vi "DCC_set_mode.vi"(6 "Modul Type to Simulate":T1 items=["Hardware Modus"=0, "Simulate DCC-100"=100, "Simulate DCU- 400/800"=200], 7 "Force Use":bool, 8 "Error In":errorcluster, 11 "DLL Path":path) -> (0 "Error Out":errorcluster, 3 "DLL Path":path)   [LabVIEW 2019]
doc: "The procedure sets the specified hardware parameter. The value of the specified parameter is transferred to the internal data structures of the DLL functions and to the DCC module ‘mod_no’ ( if ‘send_to_hard’ parameter = 1 ). \nIf ‘mod_no’ = -1, the parameter is set on all active modules.\nThe new parameter value is recalculated according to the parameter limits and hardware restrictions. Furthermore, cross dependencies between different parameters are taken into account to ensure the correct hardware operation. It is recommended to read back the parameters after setting to get their real values after recalculation. \nFirst two par_id values ( 0 - ACTIVE and 1 - PCI_BUS_NO) are not allowed - return error code. The par_id values are defined in dcc_def.h file as DCC_PARAMETERS_KEYWORDS.\n\nOktober 2018\nFrank Quadt & Stefan Smietan\ninfo@becker-hickl.com"
uses:
  DCC_Controls/DCC_ModuleTypes.ctl
panel:
  # "(c) 2021 Becker & Hickl GmbH\n     All Rights Reserved."
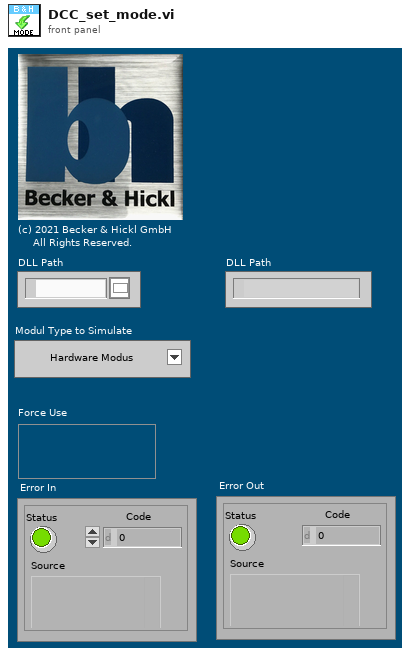
[diagram p1: front panel]
types:
  T1 = typedef "DCC_ModuleTypes.ctl" = i16
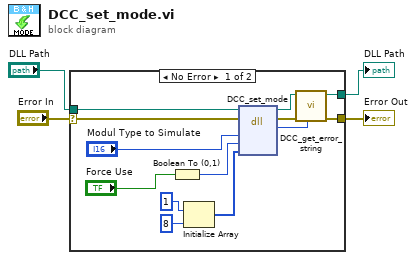
[diagram p0: block diagram]
diagram:
  n1 = case shown="No Error" "Error In" {
    selector: "Error In" -> [w17 w19]
    tunnel: [w11 w19] -> w3
    tunnel: [w13 w18] -> w2
    tunnel: "DLL Path" -> [w15 w18]
    frame No Error {
      n2 = Boolean To (0,1)(Boolean="Force Use") -> (0, 1=w14:i16)
      n3 = Initialize Array(i16 1, 8 ("dimension size")) -> (w7:i16[])
      n4 = dll-call lib="C:/Program Files/BH/DCC/DLL/dcc32.dll" fn="DCC_set_mode"(path in=w15, error in=w17, "Mode"="Modul Type to Simulate", "ForceUse"=w14, "InUse"=w7) -> (path out=w16:path, error out=w12:errorcluster, "return type"=w10:i16)  [unwired: 4 in]
      n5 = call "DCC_get_error_string.vi"("Error ID"=w10, "Error In"=w12, "DLL Path"=w16) -> ("Error Out"=w11:errorcluster, "DLL Path"=w13:path)  [unwired: 6 in, 1 out]
    }
    frame Error {
    }
  }
  "Error Out" <- w3
  "DLL Path" <- w2
